vi "WaveGenerator.vi"() -> ()   [LabVIEW 2016]
uses:
  <vilib>/measure/NI_MABase.lvlib
panel:
  in  "stop":bool
  in  "FREQ 2":dbl(knob)=1000.0 scale=0.0..100000.0
  in  "phase":dbl format="%.2p"
  out "DAC FREQ/CH, Hz":dbl
  out "String":string
  in  "STOP_RUN":bool
  in  "SIGNAL TYPE":u32(knob) scale=0.0..2.0
  in  "SIGNAL TYPE":u32(knob) scale=0.0..2.0
  in  "FREQ":dbl(knob)=1000.0 scale=0.0..100000.0
  in  "DC OFFSET":dbl(knob) scale=-5.0..5.0
  in  "AMPLITUDE":dbl(knob)=1.0 scale=0.0..5.0
  in  "DC OFFSET":dbl(knob) scale=-5.0..5.0
  in  "AMPLITUDE":dbl(knob)=1.0 scale=0.0..5.0
  # "CHANNEL A"
  # "CHANNEL B"
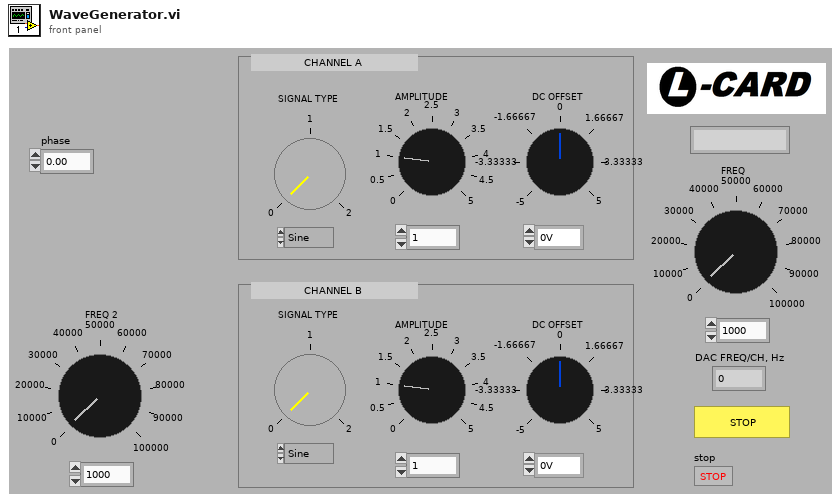
[diagram p1: front panel]
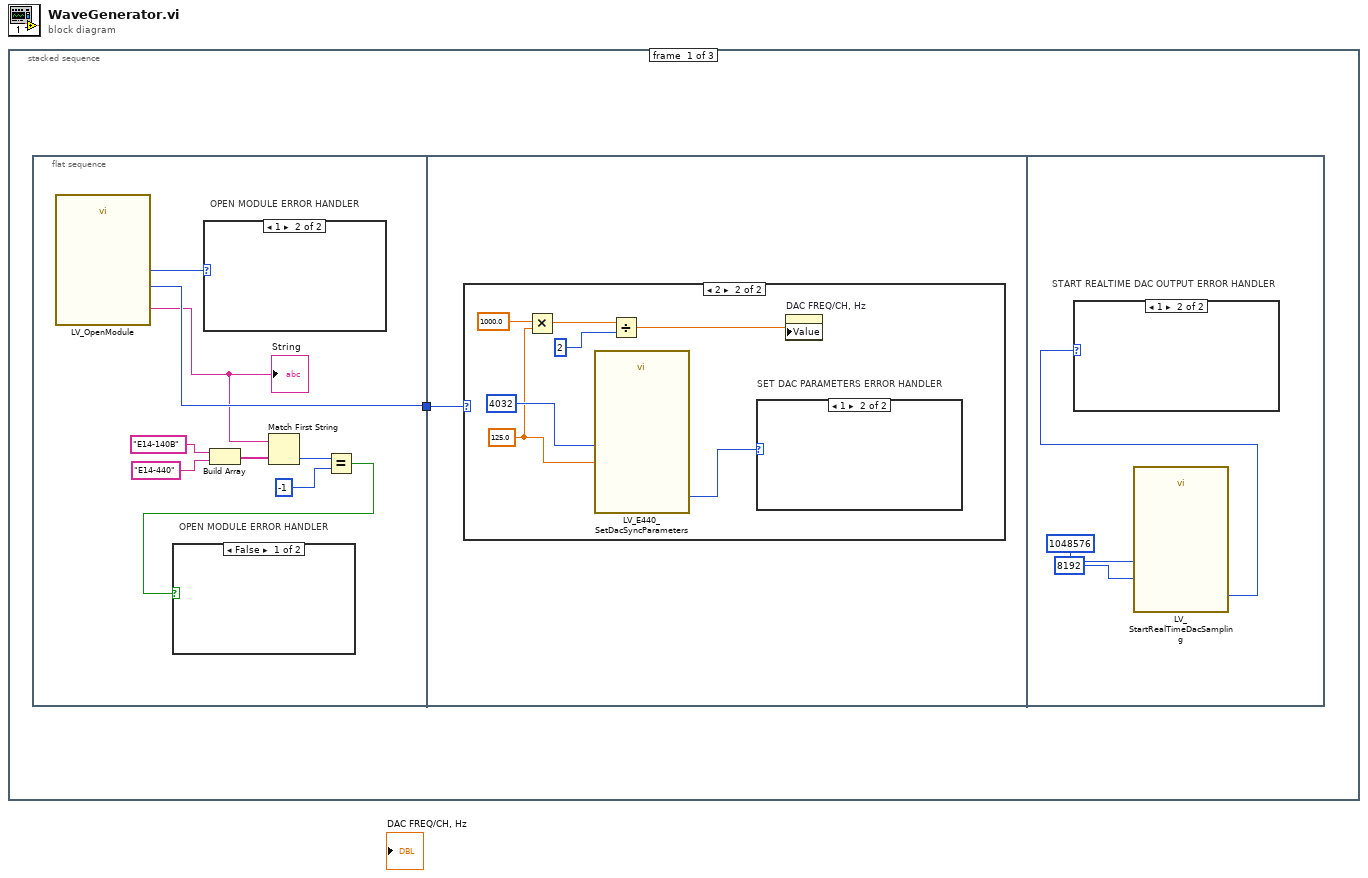
[diagram p0: block diagram]
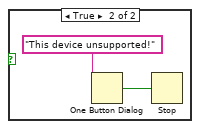
[diagram p2: hidden frame]
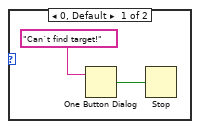
[diagram p3: hidden frame]
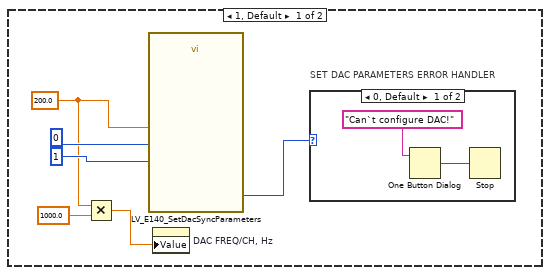
[diagram p4: hidden frame]
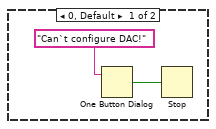
[diagram p6: hidden frame]
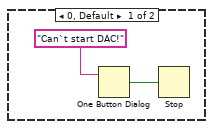
[diagram p7: hidden frame]
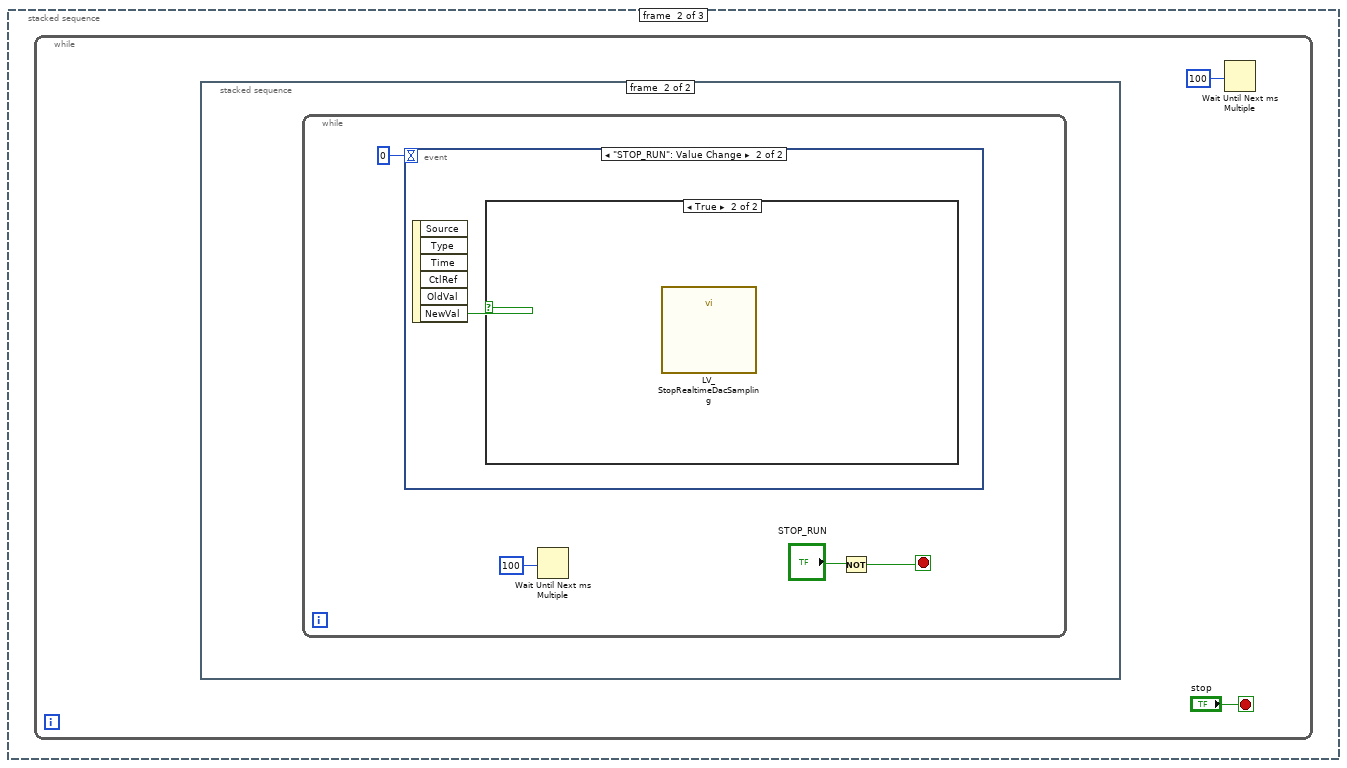
[diagram p8: hidden frame]
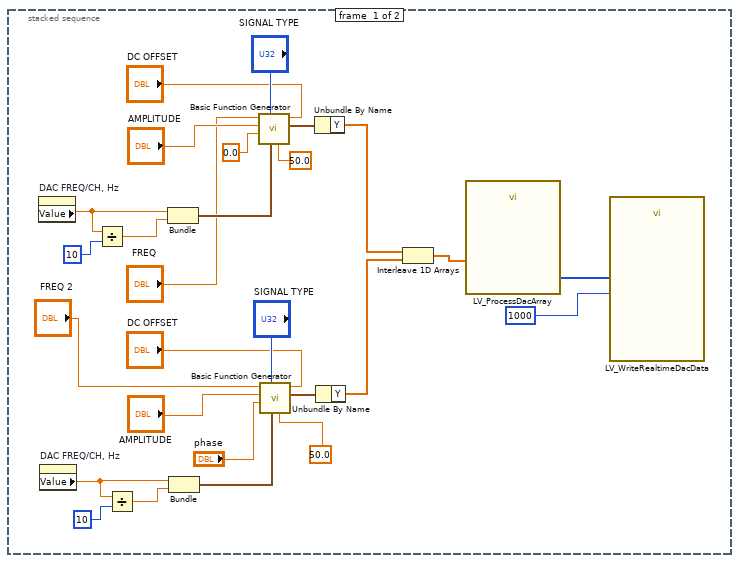
[diagram p9: hidden frame]
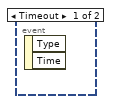
[diagram p10: hidden frame]
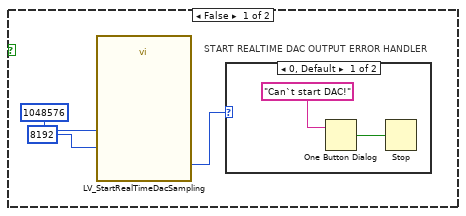
[diagram p11: hidden frame]
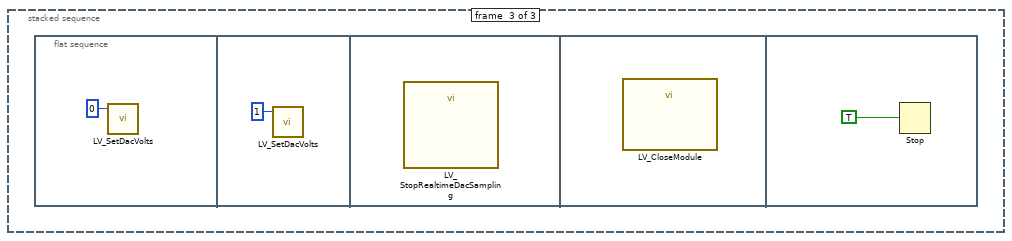
[diagram p13: hidden frame]
diagram:
  n1 = stacked-sequence {
    frame #0 {
      n2 = flat-sequence {
        tunnel: [w3] -> w1
        tunnel: w1 -> [w15]
        frame #0 {
          n3 = call <instrlib>:"LV_OpenModule.vi"() -> ("Module Name"=w2:string, "Module id"=w3:u8, "Error"=w4:u8)
          "String" <- w2
          n4 = case "OPEN MODULE ERROR HANDLER" shown="1" w4 {
            frame 0, Default {
              n5 = One Button Dialog(message="Can`t find target!") -> (true=w13:bool)  [unwired: 1 in]
              n6 = Stop(stop? (T)=w13) -> ()
            }
            frame 1 {
            }
          }
          n7 = Build Array("E14-140B", "E14-440") -> (w8:string[])
          n8 = Match First String(2:w8, 3:w2) -> (0:w7:i32)  [unwired: 1 out]
          n9 = Equal?(x=w7, y=-1) -> (x = y?=w5:bool)
          n10 = case "OPEN MODULE ERROR HANDLER" shown="False" w5 {
            frame False {
            }
            frame True {
              n11 = One Button Dialog(message="This device unsupported!") -> (true=w12:bool)  [unwired: 1 in]
              n12 = Stop(stop? (T)=w12) -> ()
            }
          }
        }
        frame #1 {
          n13 = case shown="2" w15 {
            frame 1, Default {
              w16 = 200.0
              n14 = Multiply(x=w16, y=1000.0) -> (x*y=w18:dbl)
              n15 = call <instrlib>:"LV_E140_SetDacSyncParameters.vi"("Zero on stop"=1, "Sync with ADC"=0, "Rate"=w16) -> ("Error"=w19:u32)  [unwired: 1 out]
              n16 = property on="DAC FREQ/CH, Hz" class="DigNum (strict)"("Value"=w18) -> ()  [unwired: 2 in, 2 out]
              n17 = case "SET DAC PARAMETERS ERROR HANDLER" shown="0, Default" w19 {
                frame 0, Default {
                  n18 = One Button Dialog(message="Can`t configure DAC!") -> (true=w22:bool)  [unwired: 1 in]
                  n19 = Stop(stop? (T)=w22) -> ()
                }
                frame 1 {
                }
              }
            }
            frame 2 {
              w25 = 125.0
              n20 = Multiply(x=1000.0, y=w25) -> (x*y=w26:dbl)
              n21 = call <instrlib>:"LV_E440_SetDacSyncParameters.vi"("Fifo length"=4032, "Rate"=w25) -> ("Error"=w27:u32)  [unwired: 1 out]
              n22 = Divide(x=w26, y=2) -> (x/y=w30:dbl)
              n23 = case "SET DAC PARAMETERS ERROR HANDLER" shown="1" w27 {
                frame 0, Default {
                  n24 = One Button Dialog(message="Can`t configure DAC!") -> (true=w31:bool)  [unwired: 1 in]
                  n25 = Stop(stop? (T)=w31) -> ()
                }
                frame 1 {
                }
              }
              n26 = property on="DAC FREQ/CH, Hz" class="DigNum (strict)"("Value"=w30) -> ()  [unwired: 2 in, 2 out]
            }
          }
        }
        frame #2 {
          n27 = call <instrlib>:"LV_StartRealTimeDacSampling.vi"("Packet size"=8192, "Buffer Size"=1048576) -> ("Error"=w33:u8)
          n28 = case "START REALTIME DAC OUTPUT ERROR HANDLER" shown="1" w33 {
            frame 0, Default {
              n29 = One Button Dialog(message="Can`t start DAC!") -> (true=w36:bool)  [unwired: 1 in]
              n30 = Stop(stop? (T)=w36) -> ()
            }
            frame 1 {
            }
          }
        }
      }
    }
    frame #1 {
      n31 = while {
        stop <- "stop" stop-if-true
        n32 = stacked-sequence {
          frame #0 {
            n33 = property on="DAC FREQ/CH, Hz" class="DigNum (strict)"() -> ("Value"=w45:dbl)  [unwired: 2 in, 2 out]
            n34 = property on="DAC FREQ/CH, Hz" class="DigNum (strict)"() -> ("Value"=w49:dbl)  [unwired: 2 in, 2 out]
            n35 = Divide(x=w45, y=10) -> (x/y=w44:dbl)
            n36 = Divide(x=w49, y=10) -> (x/y=w48:dbl)
            n37 = Bundle("Value"=w45, w44) -> (w65:cluster{"Value":dbl, dbl})  [unwired: 1 in]
            n38 = Bundle("Value"=w49, w48) -> (w59:cluster{"Value":dbl, dbl})  [unwired: 1 in]
            n39 = call <vilib>:"Basic Function Generator.vi"("offset"="DC OFFSET", "square wave duty cycle (%)"=50.0, "sampling info"=w65, "signal type"="SIGNAL TYPE", "phase"=sgl 0.0, "amplitude"="AMPLITUDE", "frequency"="FREQ") -> ("signal out"=w64:waveform(dbl))  [unwired: 2 in, 2 out]
            n40 = call <vilib>:"Basic Function Generator.vi"("offset"="DC OFFSET", "square wave duty cycle (%)"=50.0, "sampling info"=w59, "signal type"="SIGNAL TYPE", "phase"="phase", "amplitude"="AMPLITUDE", "frequency"="FREQ 2") -> ("signal out"=w58:waveform(dbl))  [unwired: 2 in, 2 out]
            n41 = Unbundle By Name(w64) -> ("Y"=w52:dbl[])
            n42 = Unbundle By Name(w58) -> ("Y"=w51:dbl[])
            n43 = Interleave 1D Arrays(w52, w51) -> (w50:dbl[])
            n44 = call <instrlib>:"LV_ProcessDacArray.vi"("Input data"=w50) -> ("Output data"=w43:i16[])
            n45 = call <instrlib>:"LV_WriteRealtimeDacData.vi"("Timeout"=1000, "Data"=w43) -> ()  [unwired: 2 in, 3 out]
          }
          frame #1 {
            n46 = while {
              stop <- w67 stop-if-true
              n47 = event shown="[1] \"STOP_RUN\": Value Change" {
                selector: _ -> [_ _]
                dyn-events: _ -> [_ _]
                timeout: 0 -> [_ _]
                event Timeout {
                  n48 = event-data() -> ()  [unwired: 1 in, 2 out]
                }
                event "STOP_RUN": Value Change {
                  n49 = event-data() -> ("NewVal"=w71:bool)  [unwired: 1 in, 5 out]
                  n50 = case shown="True" w71 {
                    frame False {
                      n51 = call <instrlib>:"LV_StartRealTimeDacSampling.vi"("Packet size"=8192, "Buffer Size"=1048576) -> ("Error"=w72:u8)
                      n52 = case "START REALTIME DAC OUTPUT ERROR HANDLER" shown="0, Default" w72 {
                        frame 0, Default {
                          n53 = One Button Dialog(message="Can`t start DAC!") -> (true=w75:bool)  [unwired: 1 in]
                          n54 = Stop(stop? (T)=w75) -> ()
                        }
                        frame 1 {
                        }
                      }
                    }
                    frame True {
                      n55 = call <instrlib>:"LV_StopRealtimeDacSampling.vi"() -> ()  [unwired: 1 in]
                    }
                  }
                }
              }
              n56 = Wait Until Next ms Multiple(millisecond multiple=100) -> ()  [unwired: 1 out]
              n57 = Not(x="STOP_RUN") -> (.not. x?=w67:bool)
            }
          }
        }
        n58 = Wait Until Next ms Multiple(millisecond multiple=100) -> ()  [unwired: 1 out]
      }
    }
    frame #2 {
      n59 = flat-sequence {
        frame #0 {
          n60 = call <instrlib>:"LV_SetDacVolts.vi"("Channel Num"=u32 0) -> ()  [unwired: 2 in]
        }
        frame #1 {
          n61 = call <instrlib>:"LV_SetDacVolts.vi"("Channel Num"=u32 1) -> ()  [unwired: 2 in]
        }
        frame #2 {
          n62 = call <instrlib>:"LV_StopRealtimeDacSampling.vi"() -> ()  [unwired: 1 in]
        }
        frame #3 {
          n63 = call <instrlib>:"LV_CloseModule.vi"() -> ()  [unwired: 1 in]
        }
        frame #4 {
          n64 = Stop(stop? (T)=TRUE) -> ()
        }
      }
    }
  }
